vi "OptoSpike Counter.vi"() -> ()   [LabVIEW 2017]
uses:
  Parameters for Optic Stimulation.ctl
  OptoSpike Cluster.ctl
  <vilib>/Analysis/NI_AALPro.lvlib
panel:
  out "Pooled Summary Table":string="1\t10\t100\n2\t11\t110\n3\t12\t120\n4\t13\t130\n5\t14\t140\n6\t15\t150\n7\t16\t160\n8\t17\t170\n9\t18\t180\n"
  in  "PSTH parameters":T1={"max"=0.03, "min"=0.0, "Number of bins"=50} {"min" format="%0.2f"; "max" format="%0.2f"}
  out "Histogram Graph":T2(graph) caption="PSTH"
  out "Raster plot":cluster{dbl[], dbl[]}(graph)
  in  "Optic stimulation parameters":T3={"Begin (sec)"="0.51232", "Frequency (Hz)"="10", "Epoch"="12", "Time window (ms)"="30"}
  out "[Pooled ISI] For exporting":string="1\t10\t100\n2\t11\t110\n3\t12\t120\n4\t13\t130\n5\t14\t140\n6\t15\t150\n7\t16\t160\n8\t17\t170\n9\t18\t180\n"
  out "[Raster Plot] For exporting":string="1\t10\t100\n2\t11\t110\n3\t12\t120\n4\t13\t130\n5\t14\t140\n6\t15\t150\n7\t16\t160\n8\t17\t170\n9\t18\t180\n"
  in  "Threshold (mV)":dbl=-20.0 format="%#_13g"
  in  "Load":bool
  in  "Folder Path":path=path "C:/Users/KimYG/Desktop" caption="Path of Folder"
  in  "Search Pattern":string="PV_KO_#0?.abf"
  in  "Folders to Exclude":string[](array[string]) caption="Folders to exclude"
  out "Query result":string[][](table)
  out "ISI":T2(graph) caption="히스토그램 그래프"
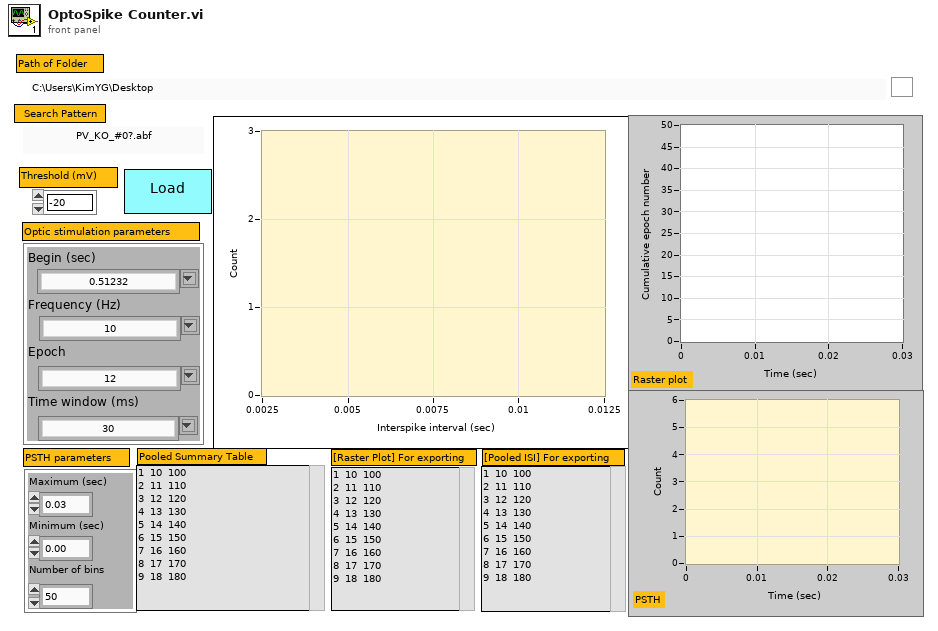
[diagram p1: front panel]
types:
  T1 = cluster{"max":dbl, "min":dbl, "Number of bins":i32}
  T2 = cluster{"X Values":dbl[], "Histogram: h(x)":i32[]}
  T3 = typedef "Parameters for Optic Stimulation.ctl" = cluster{"Begin (sec)":string, "Frequency (Hz)":string, "Epoch":string, "Time window (ms)":string}
  T4 = typedef "OptoSpike Cluster.ctl" = cluster{"File Paramters":cluster{"File Path":path, "Cell ID":string, "File Name":string, "Total Length":i32, "Trial Length (ms)":dbl, "Sweep Number":dbl, "Sampling rate":dbl}, "Raster Plot":cluster{"location":dbl[], "Sweep":i32[]}[], "Summary Table":string[][], "Pooled ISI":dbl[]}
  T5 = cluster{"File Path":path, "Cell ID":string, "File Name":string, "Total Length":i32, "Trial Length (ms)":dbl, "Sweep Number":dbl, "Sampling rate":dbl}
  T6 = enum32{"invalid app kind", "Development System", "Run Time System", "Student Edition", "Embedded LabVIEW", "Evaluation", "Custom"}
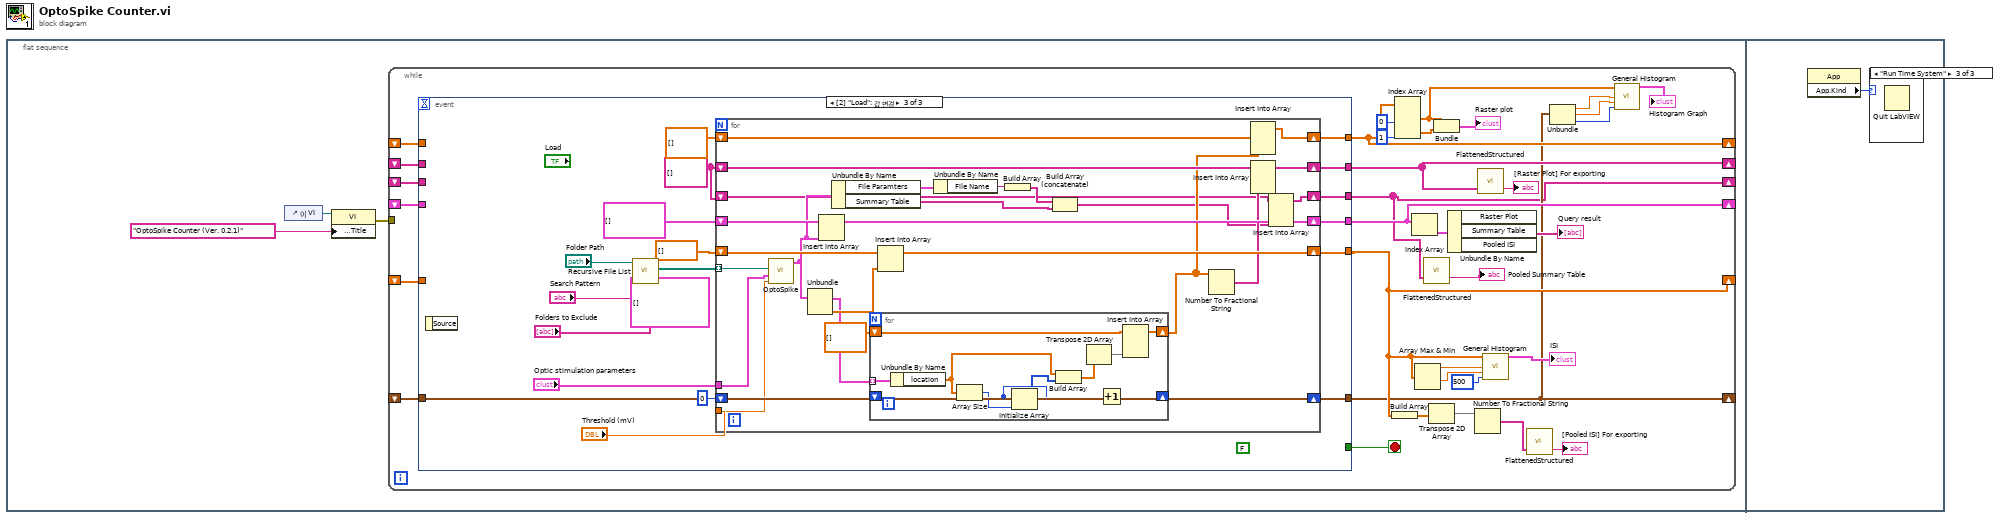
[diagram p0: block diagram]
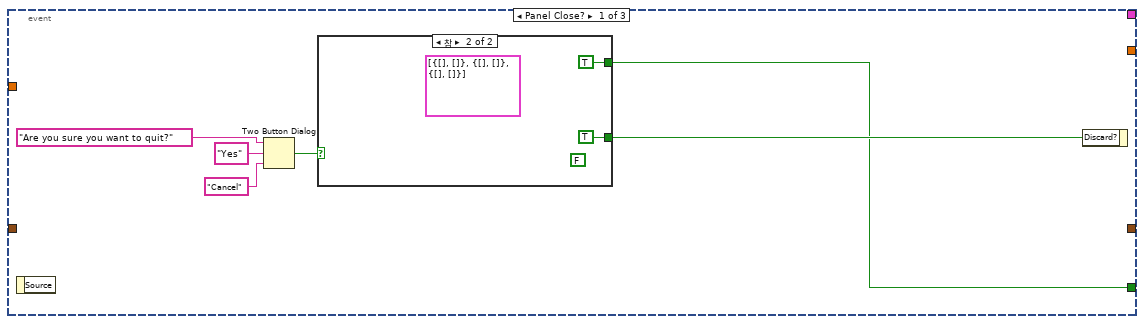
[diagram p2: hidden frame]
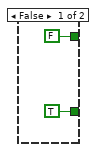
[diagram p3: hidden frame]
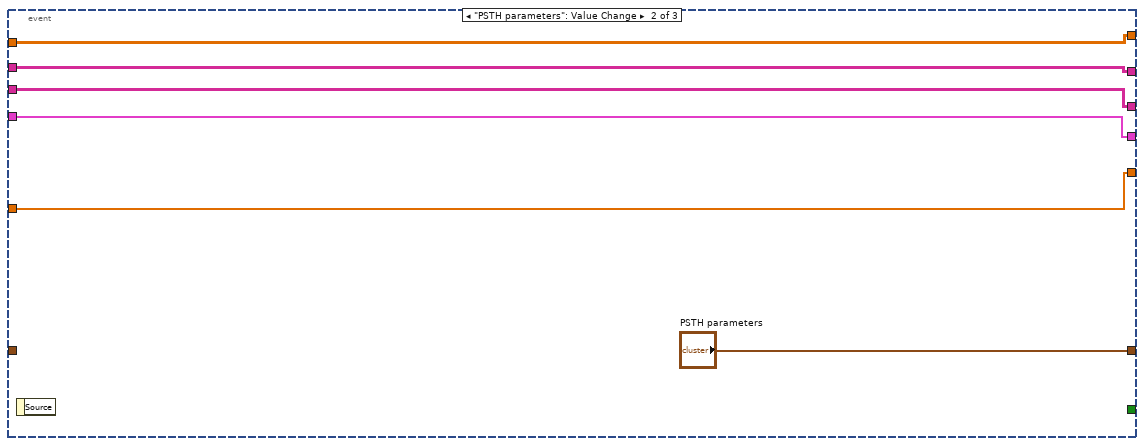
[diagram p4: hidden frame]
diagram:
  n1 = flat-sequence {
    frame #0 {
      n2 = control-ref of="이 VI"() -> (w3:refnum<vi>)
      n3 = property class="VI"(reference=w3, "Front Panel.Title"="OptoSpike Counter (Ver. 0.2.1)" ("프런트패널 윈도우:제목")) -> (error out=w1:errorcluster)  [unwired: 1 in, 1 out]
      n4 = while {
        tunnel: w1 -> [_]
        shift-right: [w30] -> _
        shift-left: _ -> [w29]
        shift-right: [w17] -> _
        shift-left: _ -> [w12]
        shift-right: [w16] -> _
        shift-left: _ -> [w13]
        shift-right: [w15] -> _
        shift-left: _ -> [w14]
        shift-right: [w11] -> _
        shift-left: _ -> [w7]
        shift-right: [w5] -> _
        shift-left: _ -> [w4]
        stop <- w37 stop-if-true
        n5 = event shown="[2] \"Load\": 값 변경" {
          selector: _ -> [_ _ _]
          dyn-events: _ -> [_ _ _]
          timeout: _ -> [_ _ _]
          tunnel: [w38 _ _] -> w37
          tunnel: [_ w51 w65] -> w30
          tunnel: w29 -> [_ w51 _]
          tunnel: [_ w50 w62] -> w17
          tunnel: [_ w52 w61] -> w16
          tunnel: [_ w53 w57] -> w15
          tunnel: w14 -> [_ w53 _]
          tunnel: w13 -> [_ w52 _]
          tunnel: w12 -> [_ w50 _]
          tunnel: [_ "PSTH parameters" w56] -> w11
          tunnel: w7 -> [_ _ w56]
          tunnel: [_ w48 w55] -> w5
          tunnel: w4 -> [_ w48 _]
          event Panel Close? {
            n6 = event-data() -> ()  [unwired: 1 in, 1 out]
            n7 = Two Button Dialog(message="Are you sure you want to quit?" ("메시지"), 1:"Cancel" ("거짓 버튼 이름(\"취소\")"), 2:"Yes" ("참 버튼 이름(\"확인\")")) -> (T button?=w40:bool)
            n8 = case shown="참" w40 {
              tunnel: [TRUE ("버림?") TRUE ("버림?")] -> w39
              tunnel: [FALSE ("버림?") TRUE ("버림?")] -> w38
              frame False {
              }
              frame True {
                (unwired) FALSE ("보이기")
                (unwired) cluster{dbl[], dbl[]}[] [{[], []}, {[], []}, {[], []}] ("Mean frequency")
              }
            }
            n9 = event-data("Discard?"=w39) -> ()  [unwired: 1 in, 1 out]
          }
          event "PSTH parameters": Value Change {
            n10 = event-data() -> ()  [unwired: 1 in, 1 out]
          }
          event "Load": Value Change {
            w54 = string[][] []
            (unwired) cluster{"location":dbl[], dbl[]}[] []
            (unwired) FALSE ("보이기")
            n11 = event-data() -> ()  [unwired: 1 in, 1 out]
            n12 = call <vilib>:"Recursive File List.vi"("Folders to Exclude"="Folders to Exclude", "pattern"="Search Pattern", "Folder Path"="Folder Path") -> ("All Files in Dir"=w67:path[])  [unwired: 4 in, 4 out]
            n13 = for {
              tunnel: w67 -> [w96] mode=indexing
              shift-right: [w91] -> w65
              shift-left: T4[] [] -> [w95]
              tunnel: "Threshold (mV)" -> [w94]
              shift-right: [w93] -> w62
              shift-left: dbl[] [] -> [w92]
              shift-right: [w89] -> w61
              shift-left: w54 -> [w88]
              tunnel: "Optic stimulation parameters" -> [w87]
              shift-right: [w83] -> _
              shift-left: 0 -> [w82]
              shift-right: [w80] -> w57
              shift-left: dbl[][] [] -> [w79]
              shift-right: [w73] -> w55
              shift-left: w54 -> [w72]
              n14 = call "OptoSpike.vi"("Threshold (mV)"=w94, "Parameters for Optic stimulation"=w87, "Path of ABF file"=w96) -> ("OptoSpike Cluster OUT"=w78:T4)  [unwired: 8 in]
              n15 = Unbundle(w78) -> ("Raster Plot"=w86:cluster{"location":dbl[], "Sweep":i32[]}[], "Pooled ISI"=w90:dbl[])  [unwired: 2 out]
              n16 = Insert Into Array(array=w95, new element=w78) -> (w91:T4[])  [unwired: 1 in]
              n17 = Unbundle By Name(w78) -> ("File Paramters"=w77:T5, "Summary Table"=w74:string[][])
              n18 = for {
                tunnel: w86 -> [w106] mode=indexing
                shift-right: [w105] -> w81
                shift-left: dbl[][] [] -> [w104]
                shift-right: [w100] -> w83
                shift-left: w82 -> [w99]
                n19 = Unbundle By Name(w106) -> ("location"=w97:dbl[])
                n20 = Array Size(array=w97) -> (size(s)=w103:i32)
                n21 = Initialize Array(w99, w103) -> (w98:i32[])
                n22 = Build Array(w97, w98) -> (w102:dbl[][])
                n23 = Transpose 2D Array(2D array=w102) -> (transposed array=w101:dbl[][])
                n24 = Increment(x=w99) -> (x+1=w100:i32)
                n25 = Insert Into Array(array=w104, new element=w101) -> (w105:dbl[][])  [unwired: 2 in]
              }
              n26 = Insert Into Array(array=w92, new element=w90) -> (w93:dbl[])  [unwired: 1 in]
              n27 = Unbundle By Name(w77) -> ("File Name"=w76:string)
              n28 = Build Array(w76) -> (w75:string[])
              n29 = Build Array (concatenate)(w75, w74) -> (w71:string[][])
              n30 = Number To Fractional String(number=w81) -> (F-format string=w85:string[][])  [unwired: 3 in]
              n31 = Insert Into Array(array=w79, new element=w81) -> (w80:dbl[][])  [unwired: 2 in]
              n32 = Insert Into Array(array=w88, new element=w85) -> (w89:string[][])  [unwired: 2 in]
              n33 = Insert Into Array(array=w72, new element=w71) -> (w73:string[][])  [unwired: 2 in]
            }
          }
        }
        n34 = Build Array(w17) -> (w28:dbl[][])
        n35 = Index Array(array=w15, index (col) #1=0 ("비활성화된 인덱스 (열)"), index (col) #2=1 ("인덱스 (열)")) -> (element #1=w19:dbl[], element #2=w21:dbl[])  [unwired: 2 in]
        n36 = Index Array(array=w30) -> (element=w32:T4)  [unwired: 1 in]
        n37 = Array Max & Min(array=w17) -> (max value=w34:dbl, min value=w35:dbl)  [unwired: 2 out]
        n38 = call <userlib>:"FlattenedStructured.vi"("Input (structured)"=w5) -> ("Output (flattened)"=→"Pooled Summary Table":string)  [unwired: 1 in, 1 out]
        n39 = Transpose 2D Array(2D array=w28) -> (transposed array=w27:dbl[][])
        n40 = Bundle(w19, w21) -> (→"Raster plot":cluster{dbl[], dbl[]})  [unwired: 1 in]
        n41 = Unbundle By Name(w32) -> ("Summary Table"=→"Query result":string[][])  [unwired: 2 out]
        n42 = Number To Fractional String(number=w27) -> (F-format string=w26:string[][])  [unwired: 3 in]
        n43 = call <userlib>:"FlattenedStructured.vi"("Input (structured)"=w16) -> ("Output (flattened)"=→"[Raster Plot] For exporting":string)  [unwired: 1 in, 1 out]
        n44 = call <vilib>:"General Histogram.vi"("X"=w17, "max"=w34, "min"=w35, "# bins"=500) -> ("Histogram Graph"=→"ISI":T2)  [unwired: 7 in, 4 out]
        n45 = call <userlib>:"FlattenedStructured.vi"("Input (structured)"=w26) -> ("Output (flattened)"=→"[Pooled ISI] For exporting":string)  [unwired: 1 in, 1 out]
        n46 = Unbundle(w11) -> ("max"=w10:dbl, "min"=w9:dbl, "Number of bins"=w8:i32)
        n47 = call <vilib>:"General Histogram.vi"("X"=w19, "max"=w10, "min"=w9, "# bins"=w8) -> ("Histogram Graph"=→"Histogram Graph":T2)  [unwired: 7 in, 4 out]
      }
    }
    frame #1 {
      n48 = property class="App"() -> ("App.Kind"=w107:T6)  [unwired: 2 in, 2 out]
      n49 = case shown="\"Run Time System\"" w107 {
        frame "invalid app kind", Default {
        }
        frame "Development System" {
        }
        frame "Run Time System" {
          n50 = Quit LabVIEW() -> ()  [unwired: 1 in]
        }
      }
    }
  }
